vi "Analog Pulse Generation.vi"() -> ()   [LabVIEW 2019, in "SubVIs.lvlib" / "Tachometer VI.lvlib"]
uses:
  Tachometer VI.lvlib
  <vilib>/Analysis/NI_AALBase.lvlib
panel:
  out "output waveform":waveform(dbl)
  in  "Sample Number":dbl=1000.0
  in  "Sample Rate":dbl=1000.0 format="%.2p"
  out "Waveform Graph 2":waveform(dbl)(graph)
  out "Waveform Chart 5":waveform(dbl)(graph)
  in  "frequency":dbl=0.0078125 format="%f"
  in  "amplitude 2":dbl=1.0 format="%0.2f"
  in  "duty cycle (%) 2":dbl=50.0 format="%0.2f"
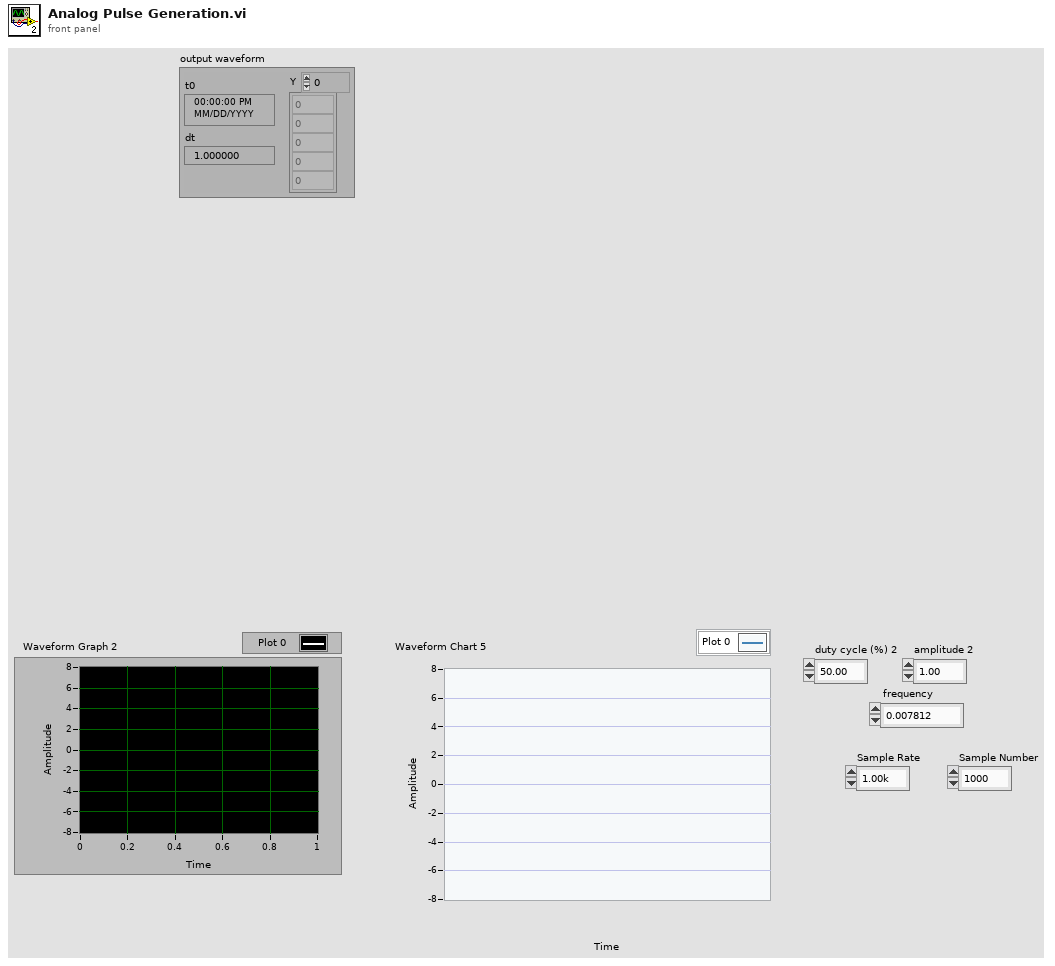
[diagram p1: front panel]
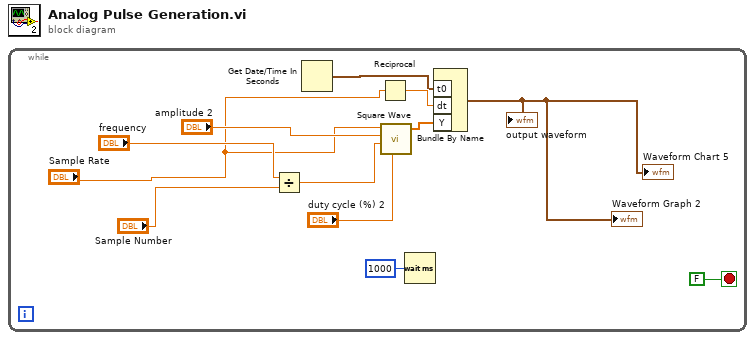
[diagram p0: block diagram]
diagram:
  n1 = while {
    stop <- FALSE stop-if-true
    n2 = Divide(x="frequency", y="Sample Number") -> (x/y=w2:dbl)
    n3 = Get Date/Time In Seconds() -> (seconds since 1Jan1904=w8:timestamp)
    n4 = Reciprocal(x="Sample Rate") -> (1/x=w9:dbl)
    n5 = call <vilib>:"Square Wave.vi"("samples"="Sample Rate", "amplitude"="amplitude 2", "frequency"=w2, "duty cycle (%)"="duty cycle (%) 2") -> ("square wave"=w7:dbl[])  [unwired: 2 in, 2 out]
    n6 = Wait (ms)(milliseconds to wait=u32 1000) -> ()  [unwired: 1 out]
    n7 = Bundle By Name("t0"=w8, "dt"=w9, "Y"=w7) -> (→"Waveform Chart 5" →"Waveform Graph 2" →"output waveform":waveform(dbl))  [unwired: 1 in]
  }
